vi "cts rts play.vi"() -> ()   [LabVIEW 2013]
uses:
  NanoArduino/NanoCmds.ctl
panel:
  out "CTS asserted?2":bool
  out "CTS asserted?1":bool
  in  "flow control (0:none)":u16(ring) items=["None", "XON/XOFF", "RTS/CTS", "XON/XOFF & RTS/CTS", "DTR/DSR", "XON/XOFF & DTR/DSR"]
  out "error out":errorcluster
  in  "error in (no error)":errorcluster
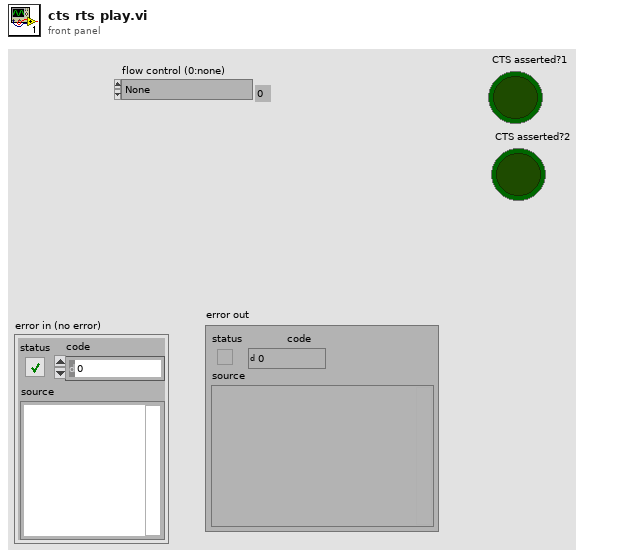
[diagram p1: front panel]
types:
  T1 = typedef "NanoCmds.ctl" = enum16{"Make digital port an output", "Make digital port an input", "Set digital pin high", "Set digital pin low", "Get digital pin state", "Get analog pin voltage", "Get analog pins difference", "Get ohms at analog pin", "Turn on current limit", "Reset Nano device", "Get digital pin state pullup", "Read current", "Initialize", "Power up uut", "Power down uut", "Get uut current draw", "Set ADC volts high", "Set ADC volts low", "Start up uut modem", "Get CTS state", "Get on_nsleep state", "Reset modem", "Get lid state", "Wait for lid closed", "Wait for lid open", "Power up, start, get curr", "Check if X2 shorted", "Power up and start up", "Check X3 shorted", "Get RTS state", "Get DTR state", "Reboot 1002759"}
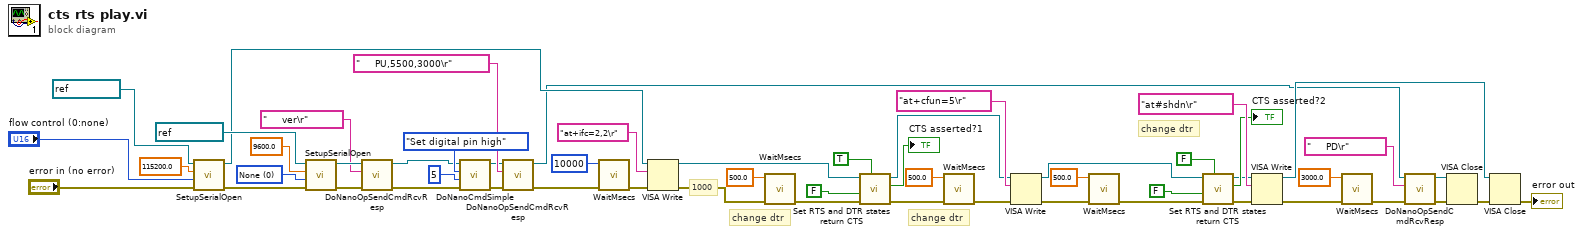
[diagram p0: block diagram]
diagram:
  w42 = u16 0 items=["None", "XON/XOFF", "RTS/CTS", "XON/XOFF & RTS/CTS", "DTR/DSR", "XON/XOFF & DTR/DSR"] ("flow control (0:none)")
  # "change dtr"
  # "change dtr"
  # "1000"
  # "change dtr"
  n1 = call "SetupSerialOpen.vi"("error in (no error)"="error in (no error)", "flow control (0:none)"="flow control (0:none)", "Baud"=115200.0, "VISA Refnum in"=refnum<visa-resource-name> "COM30" ("Modem port")) -> ("error out"=w40:errorcluster, "VISA session"=w27:refnum<visa-resource-name>)  [unwired: 6 in]
  n2 = call "SetupSerialOpen.vi"("error in (no error)"=w40, "flow control (0:none)"=w42, "Baud"=9600.0, "VISA Refnum in"=refnum<visa-resource-name> "COM21") -> ("error out"=w37:errorcluster, "VISA session"=w36:refnum<visa-resource-name>)  [unwired: 6 in]
  n3 = call "DoNanoOpSendCmdRcvResp.vi"("error in (no error)"=w37, "Cmd String"="     ver\r" ("string"), "VISA resource name"=w36) -> ("error out"=w24:errorcluster, "VISA resource name out"=w23:refnum<visa-resource-name>)  [unwired: 2 in, 5 out]
  n4 = call "DoNanoCmdSimple.vi"("error in (no error)"=w24, "Pin 1"=u32 5, "Nano Op"=NanoCmds."Set digital pin high", "VISA resource name"=w23) -> ("error out"=w21:errorcluster, "VISA resource name 2"=w22:refnum<visa-resource-name>)  [unwired: 3 in, 2 out]
  n5 = call "DoNanoOpSendCmdRcvResp.vi"("error in (no error)"=w21, "Cmd String"="     PU,5500,3000\r" ("string"), "VISA resource name"=w22) -> ("error out"=w34:errorcluster, "VISA resource name out"=w10:refnum<visa-resource-name>)  [unwired: 2 in, 5 out]
  n6 = call "WaitMsecs.vi"("error in (no error)"=w34, "Wait Msecs"=u32 10000) -> ("error out"=w28:errorcluster)  [unwired: 9 in]
  n7 = VISA Write(VISA resource name=w27, write buffer="at+ifc=2,2\r", error in (no error)=w28) -> (VISA resource name out=w11:refnum<visa-resource-name>, error out=w30:errorcluster)  [unwired: 1 out]
  n8 = call "WaitMsecs.vi"("error in (no error)"=w30, "Wait Msecs"=500.0) -> ("error out"=w12:errorcluster)  [unwired: 9 in]
  n9 = call "Set RTS and DTR states return CTS.vi"("Assert DTR?"=TRUE, "error in (no error)"=w12, "Assert RTS?"=FALSE, "VISA Refnum in"=w11) -> ("error out"=w15:errorcluster, "CTS asserted?"=→"CTS asserted?1":bool, "Visa ref out"=w14:refnum<visa-resource-name>)  [unwired: 5 in]
  n10 = call "WaitMsecs.vi"("error in (no error)"=w15, "Wait Msecs"=500.0) -> ("error out"=w13:errorcluster)  [unwired: 9 in]
  n11 = VISA Write(VISA resource name=w14, write buffer="at+cfun=5\r", error in (no error)=w13) -> (VISA resource name out=w2:refnum<visa-resource-name>, error out=w6:errorcluster)  [unwired: 1 out]
  n12 = call "WaitMsecs.vi"("error in (no error)"=w6, "Wait Msecs"=500.0) -> ("error out"=w5:errorcluster)  [unwired: 9 in]
  n13 = call "Set RTS and DTR states return CTS.vi"("Assert DTR?"=FALSE, "error in (no error)"=w5, "Assert RTS?"=FALSE, "VISA Refnum in"=w2) -> ("error out"=w4:errorcluster, "CTS asserted?"=→"CTS asserted?2":bool, "Visa ref out"=w1:refnum<visa-resource-name>)  [unwired: 5 in]
  n14 = VISA Write(VISA resource name=w1, write buffer="at#shdn\r", error in (no error)=w4) -> (VISA resource name out=w44:refnum<visa-resource-name>, error out=w48:errorcluster)  [unwired: 1 out]
  n15 = call "WaitMsecs.vi"("error in (no error)"=w48, "Wait Msecs"=3000.0) -> ("error out"=w45:errorcluster)  [unwired: 9 in]
  n16 = call "DoNanoOpSendCmdRcvResp.vi"("error in (no error)"=w45, "Cmd String"="     PD\r" ("string"), "VISA resource name"=w10) -> ("error out"=w50:errorcluster, "VISA resource name out"=w49:refnum<visa-resource-name>)  [unwired: 2 in, 5 out]
  n17 = VISA Close(VISA resource name=w49, error in (no error)=w50) -> (error out=w52:errorcluster)
  n18 = VISA Close(VISA resource name=w44, error in (no error)=w52) -> (error out=→"error out":errorcluster)
